vi "SaveData.vi"(2 "Bamp_next":dbl, 3 "path":string, 4 "index":dbl, 5 "Findex":dbl, 6 "Bmax_pos":dbl, 7 "Bamp_max":dbl, 8 "error in":errorcluster, 9 "Amax_pos":dbl, 10 "Aamp_next":dbl, 11 "Aamp_max":dbl) -> (0 "error out":errorcluster)   [LabVIEW 2015]
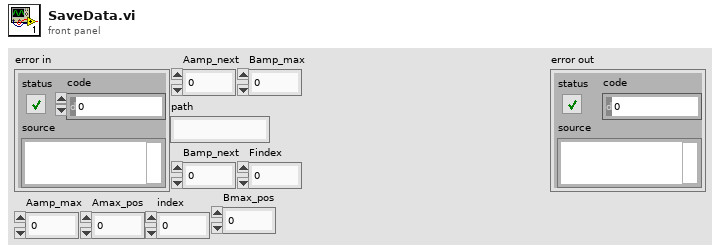
[diagram p1: front panel]
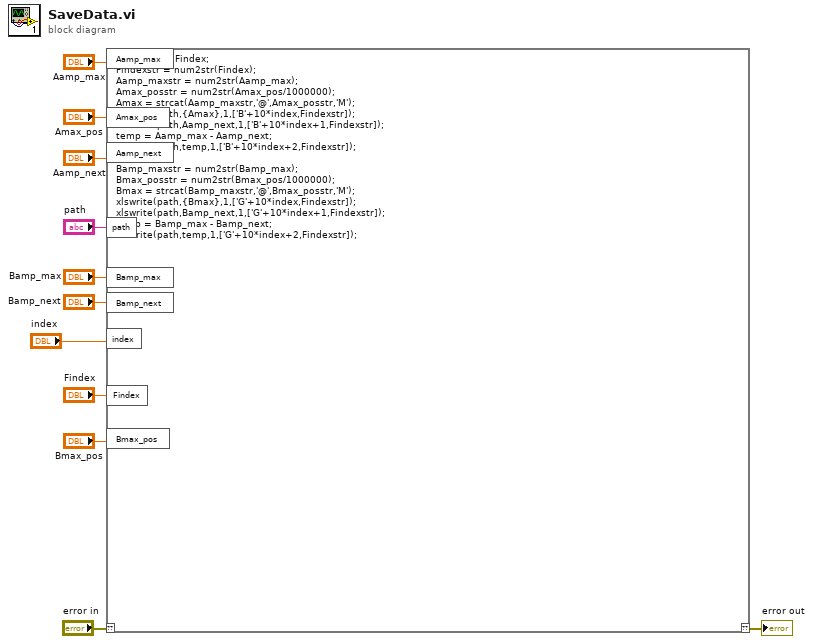
[diagram p0: block diagram]
diagram:
  n1 = script code="Findex = 5+Findex;\nFindexstr = num2str(Findex);\nAamp_maxstr = num2str(Aamp_max);\nAmax_posstr = num2str(Amax_pos/1000000);\nAmax = strcat(Aamp_maxstr,'@',Amax_posstr,'M');\nxlswrite(path,{Amax},1,['B'+10*index,Findexstr]);\nxlswrite(path,Aamp_next,1,['B'+10*index+1,Findexstr]);\ntemp = Aamp_max - Aamp_next;\nxlswrite(path,temp,1,['B'+10*index+2,Findexstr]);\n\nBamp_maxstr = num2str(Bamp_max);\nBmax_posstr = num2str(Bmax_pos/1000000);\nBmax = strcat(Bamp_maxstr,'@',Bmax_posstr,'M');\nxlswrite(path,{Bmax},1,['G'+10*index,Findexstr]);\nxlswrite(path,Bamp_next,1,['G'+10*index+1,Findexstr]);\ntemp = Bamp_max - Bamp_next;\nxlswrite(path,temp,1,['G'+10*index+2,Findexstr]);"("??"="error in", "Aamp_max"="Aamp_max", "Aamp_next"="Aamp_next", "path"="path", "index"="index", "Bamp_max"="Bamp_max", "Bamp_next"="Bamp_next", "Findex"="Findex", "Amax_pos"="Amax_pos", "Bmax_pos"="Bmax_pos") -> ("??"=→"error out":errorcluster)
